vi "_097.vi"() -> ()   [LabVIEW 2020]
panel:
  out "Iteration":i32
  out "x+y":i32
  # "What is the iteration count for while loop ?"
  # "The iteration count is zero why because 2+2=4 , in the 0'th iteration the output is 4 (in comparison operator -> Greaterthen or equal to condition is 4 & the output is 4 ) , So the condition terminal was stops the loop , So the loop will stops in the zero'th iteration and the iteration count is zero."
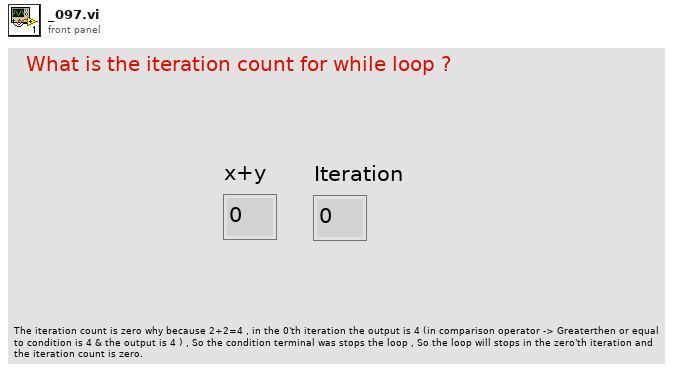
[diagram p1: front panel]
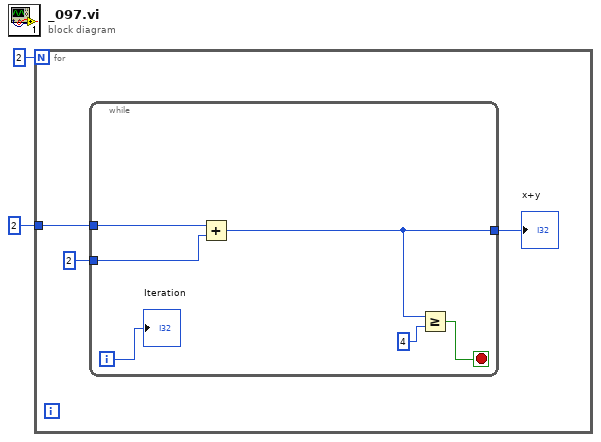
[diagram p0: block diagram]
diagram:
  n1 = for {
    N: 2 -> [_]
    tunnel: 2 -> [w3]
    n2 = while {
      tunnel: 2 -> [w11]
      tunnel: [w9] -> w4
      tunnel: w3 -> [w6]
      i -> [w7]
      stop <- w10 stop-if-true
      n3 = Add(x=w6, y=w11) -> (x+y=w9:i32)
      n4 = Greater Or Equal?(x=w9, y=4) -> (x >= y?=w10:bool)
      "Iteration" <- w7
    }
    "x+y" <- w4
  }
